vi "Pharse_Str2Param (SubVI).vi"(1 "param_ret":string) -> (0 "param":T1={"Time_sec"="7005.1", "HeadPow%"=0, "Temp (C)"=50})   [LabVIEW 2018]
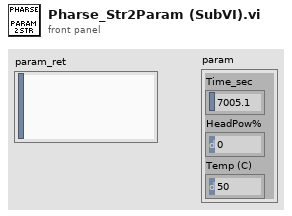
[diagram p1: front panel]
types:
  T1 = cluster{"Time_sec":string, "HeadPow%":i32, "Temp (C)":u8}
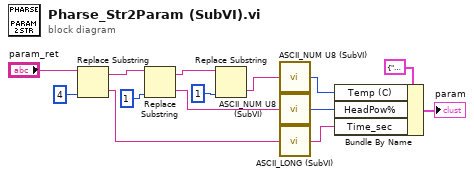
[diagram p0: block diagram]
diagram:
  n1 = Replace Substring(2:4 ("length (len. of substring)"), 5:"param_ret") -> (0:w3:string, 1:w13:string)  [unwired: 2 in]
  n2 = Replace Substring(2:1 ("length (len. of substring)"), 5:w13) -> (0:w4:string, 1:w12:string)  [unwired: 2 in]
  n3 = Replace Substring(2:1 ("length (len. of substring)"), 5:w12) -> (0:w5:string)  [unwired: 2 in, 1 out]
  n4 = call "ASCII_NUM U8 (SubVI).vi"("String"=w5) -> ("Number"=w6:i32)
  n5 = call "ASCII_NUM U8 (SubVI).vi"("String"=w4) -> ("Number"=w8:i32)
  n6 = call "ASCII_LONG (SubVI).vi"("ascii in"=w3) -> ("String out"=w7:string)
  n7 = Bundle By Name(cluster=T1 {"Time_sec"="7005.1", "HeadPow%"=0, "Temp (C)"=50} ("param"), "Temp (C)"=w6, "HeadPow%"=w8, "Time_sec"=w7) -> (→"param":T1)
